vi "Write Command.vi"(8 "error in":errorcluster, 10 "command":string, 11 "pipe in":T1) -> (0 "error out":errorcluster, 3 "pipe out":T1)   [LabVIEW 2013, in "GOLPI library.lvlib"]
doc: "Sends command to GNU Octave. End of line is added automatically if missing."
uses:
  GOLPI library.lvlib
  LV Process.lvlibp/Pipe Handle.ctl
  LV Process.lvlibp
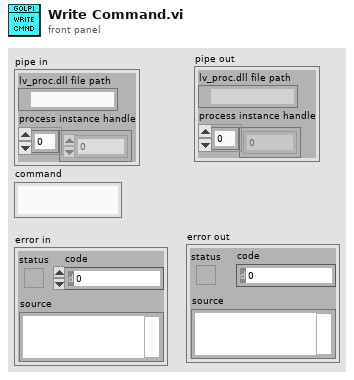
[diagram p1: front panel]
types:
  T1 = typedef "LV Process.lvlibp/Pipe Handle.ctl" = cluster{"lv_proc.dll file path":path, "process instance handle":u32[]}
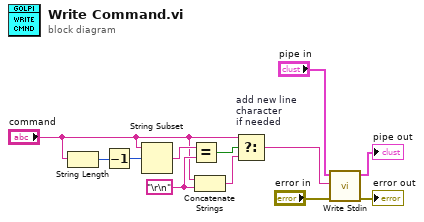
[diagram p0: block diagram]
diagram:
  w5 = "\r\n"
  n1 = String Length(string="command") -> (length=w9:i32)
  n2 = Decrement(x=w9) -> (x-1=w8:i32)
  n3 = String Subset(string="command", offset (0)=w8) -> (substring=w7:string)  [unwired: 1 in]
  n4 = Equal?(x=w7, y=w5) -> (x = y?=w6:bool)
  n5 = Concatenate Strings("command", w5) -> (w4:string)
  n6 = Select "add new line\ncharacter\nif needed"(t="command", s=w6, f=w4) -> (s? t:f=w2:string)
  n7 = call "Write Stdin.vi"("error in"="error in", "write buffer"=w2, "pipe in"="pipe in") -> ("error out"=→"error out":errorcluster, "pipe out"=→"pipe out":T1)  [unwired: 6 in, 1 out]
